vi "ReleaseLotCheck.vi"() -> ()   [LabVIEW 2012]
uses:
  <vilib>/Utility/miscctls.llb/LVDateTimeRec.ctl
  <vilib>/Utility/NIReport.llb/NI_report.lvclass
  <vilib>/addons/_office/excel.llb/Excel Get Data (str).vi
  <vilib>/addons/_office/excel.llb/Excel Get Data (i32).vi
  <vilib>/Utility/NIReport.llb/Excel/NI_Excel.lvclass
  <vilib>/addons/_office/NI_ReportGenerationToolkit.lvlib
  <vilib>/Utility/SMTP/NI_SMTPEmail.lvlib
panel:
  out "date string 3":string
  out "spreadsheet string":string
  out "data":string
  out "result":bool
  out "date string 2":string
  out "date string":string
  in  "date time rec":T1
  out "data 2":i32
  out "row":i32
  in  "start (0, 0)":cluster{"start row":i32, "start column":i32}
  out "output array":string[](array[string])
  out "step":string
  out "error out":errorcluster
  out "array":string[](array[string])
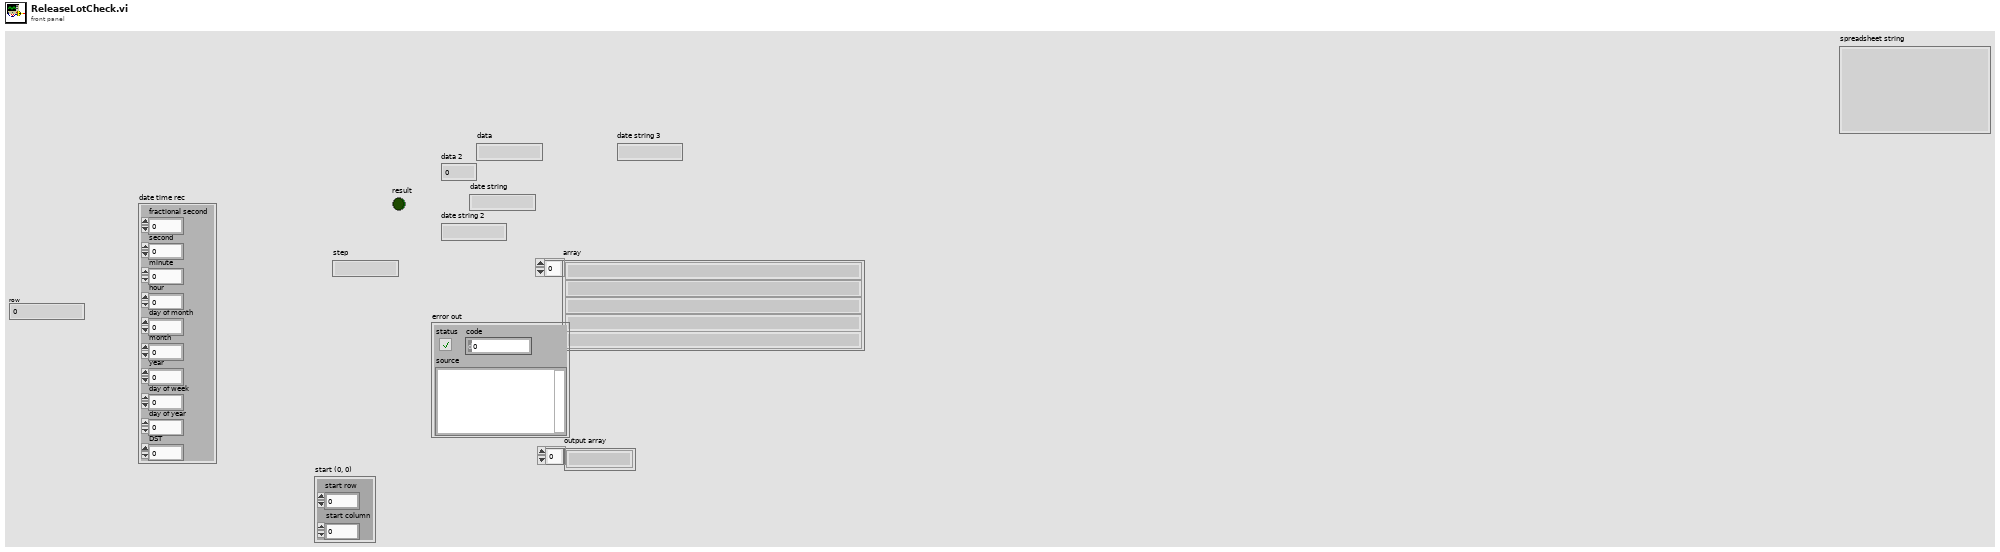
[diagram p1: front panel]
types:
  T1 = typedef "LVDateTimeRec.ctl" = cluster{"fractional second":dbl, "second":i32, "minute":i32, "hour":i32, "day of month":i32, "month":i32, "year":i32, "day of week":i32, "day of year":i32, "DST":i32}
  T2 = enum16{"Standard Report", "HTML", "Word", "Excel"}
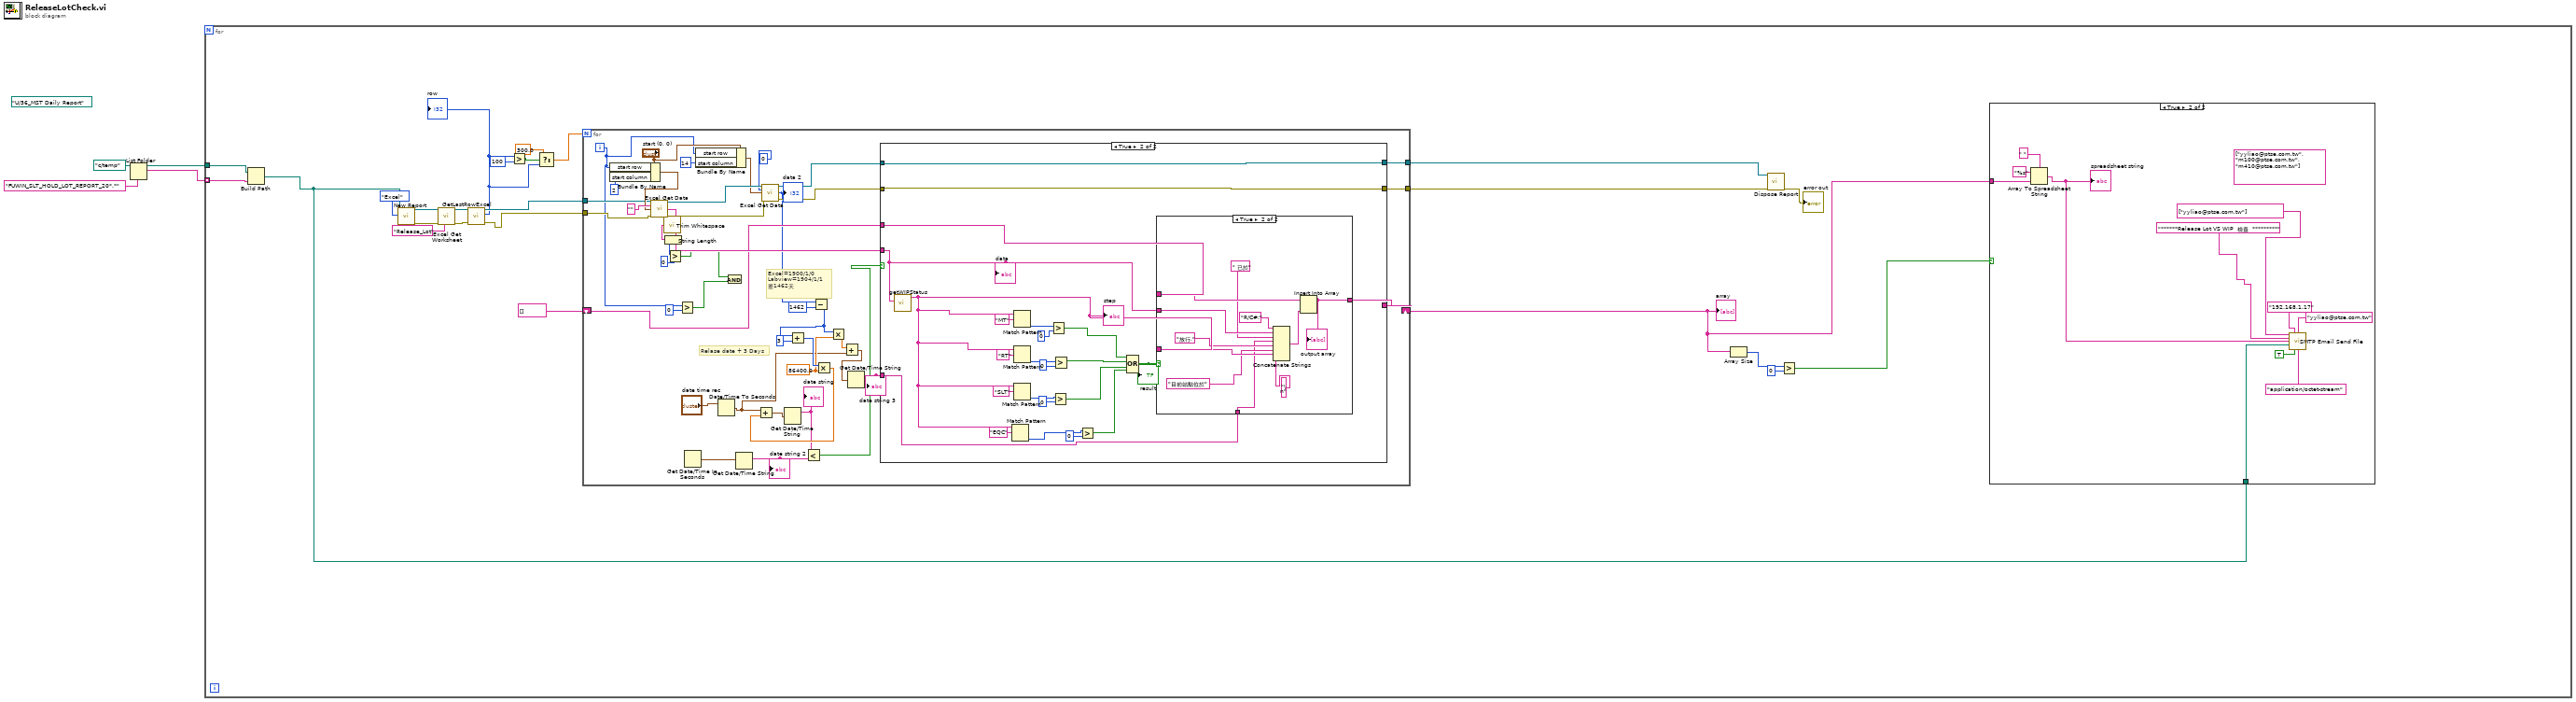
[diagram p0: block diagram]
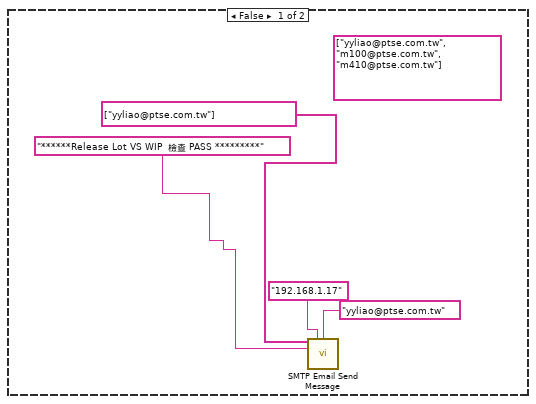
[diagram p2: hidden frame]
diagram:
  (unwired) path "U:/36_MST Daily Report" ("path")
  n1 = List Folder(path=path "c:/temp", pattern="FUWIN_SLT_HOLD_LOT_REPORT_20*.*") -> (path out=w3:path, filenames=w2:string[])  [unwired: 2 in, 2 out]
  n2 = for {
    tunnel: w3 -> [w12]
    tunnel: w2 -> [w11] mode=indexing
    n3 = Build Path(base path=w12, name or relative path=w11) -> (appended path=w5:path)
    n4 = call <vilib>:"New Report.vi"("report type"=T2."Excel" ("Report Type"), "template (empty)"=w5) -> ("report out"=w27:refnum<class "NI_report.lvclass">, "error out"=w26:errorcluster)  [unwired: 12 in]
    n5 = call <vilib>:"Excel Get Worksheet.vi"("report in"=w27, "error in (no error)"=w26, "name (\"\")"="Release_Lot" ("name (\"\")")) -> ("report out"=w25:refnum<class "NI_report.lvclass">, "error out"=w24:errorcluster)  [unwired: 11 in]
    n6 = call "GetLastRowExcel.vi"("error in (no error)"=w24, "report in"=w25) -> ("error out"=w23:errorcluster, "row"=w16:i32, "report out"=w22:refnum<class "NI_report.lvclass">)  [unwired: 7 in]
    "row" <- w16
    n7 = Greater?(x=w16, y=100) -> (0:w18:bool)
    n8 = Select(t=300.0, s=w18, f=w16) -> (s? t:f=w15:dbl)
    n9 = for {
      N: w15 -> [_]
      tunnel: w22 -> [w77]
      tunnel: w23 -> [w76]
      tunnel: [w70] -> w10
      tunnel: [w80] -> w9
      shift-right: [w72] -> w6
      shift-left: string[] [] ("array") -> [w71]
      i -> [w63]
      w48 = 86400.0 ("y")
      # "Relase date + 3 Days"
      # "Excel=1900/1/0\nLabview=1904/1/1\n差1462天"
      n10 = Bundle By Name(cluster="start (0, 0)", "start row"=w63, "start column"=2) -> (w79:cluster{"start row":i32, "start column":i32})
      n11 = call-poly <vilib>:"Excel Get Data.vi"("report in"=w77, "data type"="", "start (0, 0)"=w79, "error in (no error)"=w76) -> ("report out"=w67:refnum<class "NI_report.lvclass">, "data"=w78:string, "error out"=w69:errorcluster)  [unwired: 9 in]
      n12 = call <vilib>:"Trim Whitespace.vi"("string"=w78) -> ("trimmed string"=w82:string)  [unwired: 1 in]
      n13 = String Length(string=w82) -> (length=w81:i32)
      n14 = Greater?(x=w81, y=0) -> (0:w73:bool)
      n15 = Greater?(x=w63, y=0) -> (0:w74:bool)
      n16 = Get Date/Time In Seconds() -> (seconds since 1Jan1904=w54:timestamp)
      n17 = Bundle By Name(cluster="start (0, 0)", "start row"=w63, "start column"=14) -> (w62:cluster{"start row":i32, "start column":i32})
      n18 = Date/Time To Seconds(2:"date time rec") -> (0:w46:timestamp)  [unwired: 1 in]
      n19 = And(x=w73, y=w74) -> ()  [unwired: 1 out]
      n20 = Get Date/Time String(seconds (now)=w54) -> (date string=w51:string)  [unwired: 2 in, 1 out]
      "date string 2" <- w51
      n21 = call-poly <vilib>:"Excel Get Data.vi"("report in"=w67, "data type"=0, "start (0, 0)"=w62, "error in (no error)"=w69) -> ("report out"=w66:refnum<class "NI_report.lvclass">, "data"=w59:i32, "error out"=w68:errorcluster)  [unwired: 9 in]
      "data 2" <- w59
      n22 = Subtract(x=w59, y=1462) -> (x-y=w49:i32)
      n23 = Add(x=w49, y=3) -> (x+y=w55:i32)
      n24 = Multiply(x=w55, y=w48) -> (x*y=w58:dbl)
      n25 = Add(x=w46, y=w58) -> (x+y=w53:timestamp)
      n26 = Get Date/Time String(seconds (now)=w53) -> (date string=w52:string)  [unwired: 2 in, 1 out]
      "date string" <- w52
      n27 = Less?(x=w52, y=w51) -> (x < y?=w50:bool)
      n28 = Multiply(x=w49, y=w48) -> (x*y=w47:dbl)
      n29 = Add(x=w47, y=w46) -> (x+y=w45:timestamp)
      n30 = Get Date/Time String(seconds (now)=w45) -> (date string=w44:string)  [unwired: 2 in, 1 out]
      "date string 3" <- w44
      n31 = case shown="True" w50 {
        tunnel: w78 -> [_ w98]
        tunnel: w66 -> [w88 w112]
        tunnel: w68 -> [w87 w111]
        tunnel: [w88 w112] -> w70
        tunnel: [w87 w111] -> w80
        tunnel: [w86 w97] -> w72
        tunnel: w71 -> [w86 w96]
        tunnel: w44 -> [_ w89]
        frame False {
        }
        frame True {
          n32 = call "getWIPStatus.vi"("Lotno"=w98) -> ("step"=w91:string)  [unwired: 9 in, 1 out]
          "step" <- w91
          n33 = Match Pattern(string=w91, regular expression="EQC") -> (offset past match=w93:i32)  [unwired: 1 in, 3 out]
          n34 = Match Pattern(string=w91, regular expression="SLT") -> (offset past match=w103:i32)  [unwired: 1 in, 3 out]
          n35 = Match Pattern(string=w91, regular expression="MT") -> (offset past match=w107:i32)  [unwired: 1 in, 3 out]
          n36 = Match Pattern(string=w91, regular expression="RT") -> (offset past match=w105:i32)  [unwired: 1 in, 3 out]
          n37 = Greater?(x=w107, y=0) -> (0:w101:bool)
          n38 = Greater?(x=w103, y=0) -> (0:w99:bool)
          n39 = Greater?(x=w105, y=0) -> (0:w100:bool)
          n40 = Greater?(x=w93, y=0) -> (0:w92:bool)
          n41 = Compound Arithmetic op=OR(w101, w100, w99, w92) -> (w90:bool)
          "result" <- w90
          n42 = case shown="True" w90 {
            tunnel: w98 -> [_ w116]
            tunnel: [w113 w124] -> w97
            tunnel: w96 -> [w113 w123]
            tunnel: w91 -> [_ w120]
            tunnel: w89 -> [_ w114]
            frame False {
            }
            frame True {
              n43 = Concatenate Strings("R/C#:" ("string"), w116, " 已於" ("string"), w114, "放行," ("string"), "目前站點位於" ("string"), w120, "\n" ("string")) -> (w122:string)
              n44 = Insert Into Array(array=w123, new element=w122) -> (w124:string[])  [unwired: 1 in]
              "output array" <- w124
            }
          }
          "data" <- w98
        }
      }
    }
    "array" <- w6
    n45 = Array Size(array=w6) -> (size(s)=w14:i32)
    n46 = call-dynamic "Dispose Report.vi"("report in"=w10, "error in (no error)"=w9) -> ("error out"=→"error out":errorcluster)  [unwired: 13 in]
    n47 = Greater?(x=w14, y=0) -> (0:w7:bool)
    n48 = case shown="True" w7 {
      tunnel: w6 -> [_ w37]
      tunnel: w5 -> [_ w34]
      frame False {
        (unwired) string[] ["yyliao@ptse.com.tw", "m100@ptse.com.tw", "m410@ptse.com.tw"] ("recipients")
        n49 = call <vilib>:"SMTP Email Send Message.vi"("recipients"=string[] ["yyliao@ptse.com.tw"], "mail server"="192.168.1.17", "return address"="yyliao@ptse.com.tw", "subject ([No Subject])"="******Release Lot VS WIP  檢查 PASS *********") -> ()  [unwired: 10 in, 2 out]
      }
      frame True {
        (unwired) string[] ["yyliao@ptse.com.tw", "m100@ptse.com.tw", "m410@ptse.com.tw"] ("recipients")
        n50 = Array To Spreadsheet String(delimiter (Tab)=" ", array=w37, 3:"%s" ("format string")) -> (spreadsheet string=w36:string)
        "spreadsheet string" <- w36
        n51 = call <vilib>:"SMTP Email Send File.vi"("recipients"=string[] ["yyliao@ptse.com.tw"], "mail server"="192.168.1.17", "return address"="yyliao@ptse.com.tw", "subject ([No Subject])"="******Release Lot VS WIP  檢查  *********", "message"=w36, "file path"=w34, "binary? (F)"=TRUE, "MIME content-type (application/octet-stream)"="application/octet-stream") -> ()  [unwired: 6 in, 2 out]
      }
    }
  }
